vi "Calc FD_Frame Duration.vi"(8 "Bit Time FD (seconds)":dbl, 9 "Bit Time (seconds)":dbl, 10 "Avg.DataLength (bits)":dbl, 11 "Avg.ArbitrationLength (bits)":dbl) -> (3 "Frame.Duration(us)":u32)   [LabVIEW 2019, in "XNET-Bus-Load-Calculator.lvlib" / "CANBus_Load_Calculator.lvclass"]
uses:
  CANBus_Load_Calculator.lvclass
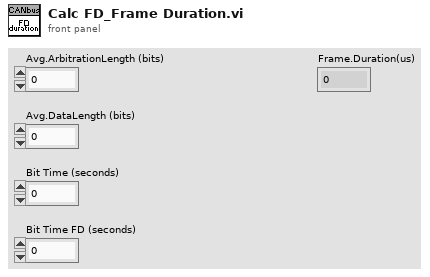
[diagram p1: front panel]
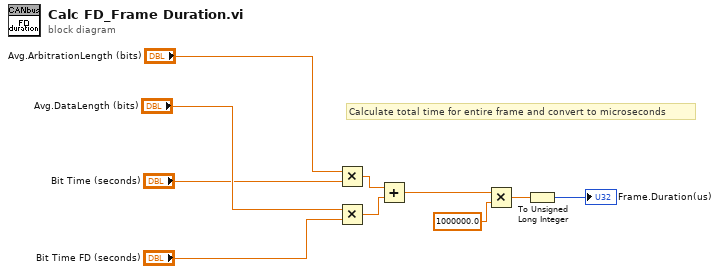
[diagram p0: block diagram]
diagram:
  # "Calculate total time for entire frame and convert to microseconds"
  n1 = Multiply(x="Avg.ArbitrationLength (bits)", y="Bit Time (seconds)") -> (x*y=w1:dbl)
  n2 = Multiply(x="Avg.DataLength (bits)", y="Bit Time FD (seconds)") -> (x*y=w2:dbl)
  n3 = Add(x=w1, y=w2) -> (x+y=w5:dbl)
  n4 = Multiply(x=w5, y=1000000.0) -> (x*y=w3:dbl)
  n5 = To Unsigned Long Integer(number=w3) -> (unsigned 32bit integer=→"Frame.Duration(us)":u32)
